vi "Shutdown.vi"(8 "error in (no error)":errorcluster, 11 "Insight in":refnum<class "Insight.lvclass">) -> (0 "error out":errorcluster, 3 "Insight out":refnum<class "Insight.lvclass">)   [LabVIEW 2014, in "Insight.lvclass"]
uses:
  Insight.lvclass
  Insight/Telnet Session.ctl
  Insight.lvclass/Insight.ctl
  Laser.lvclass
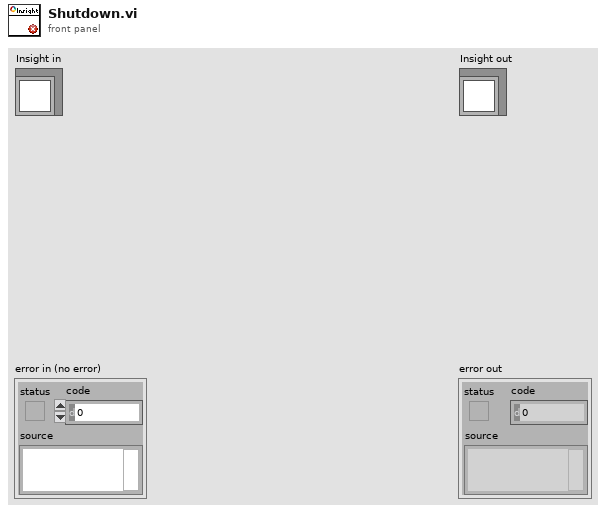
[diagram p1: front panel]
types:
  T1 = typedef "Telnet Session.ctl" = refnum<k1>
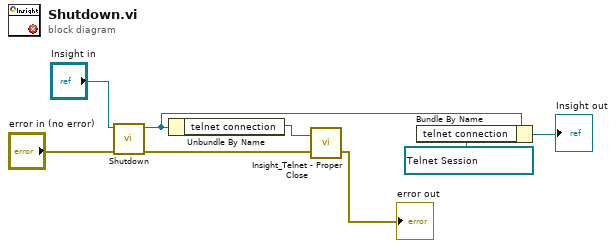
[diagram p0: block diagram]
diagram:
  w2 = T1 refnum items=["telnet connection"] ("telnet connection")
  n1 = call-parent "Shutdown.vi"("error in (no error)"="error in (no error)", "Laser in"="Insight in") -> ("error out"=w5:errorcluster, "Laser out"=w4:refnum<class "Insight.lvclass">)  [unwired: 8 in]
  n2 = Unbundle By Name(w4) -> ("telnet connection"=w6:T1)
  n3 = call "Insight_Telnet - Proper Close.vi"("error in"=w5, "telnet connection"=w6) -> ("error out"=→"error out":errorcluster)  [unwired: 1 in]
  n4 = Bundle By Name(cluster=w4, "telnet connection"=w2) -> (→"Insight out":refnum<class "Insight.lvclass">)
